vi "signalThreshold.vi"(11 "VE":dbl[](array[numeric])) -> (2 "minValue":dbl, 3 "Threshould":dbl)   [LabVIEW 2011]
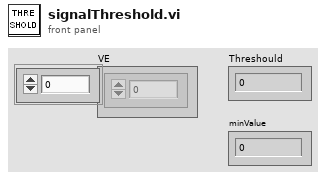
[diagram p1: front panel]
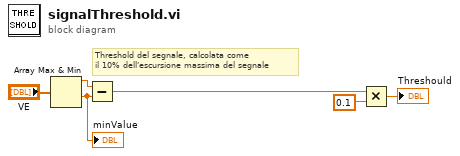
[diagram p0: block diagram]
diagram:
  # "Threshold del segnale, calcolata come\nil 10% dell'escursione massima del segnale"
  n1 = Array Max & Min(array="VE") -> (max value=w1:dbl, min value=w2:dbl)  [unwired: 2 out]
  "minValue" <- w2
  n2 = Subtract(x=w1, y=w2) -> (x-y=w3:dbl)
  n3 = Multiply(x=w3, y=0.1) -> (x*y=→"Threshould":dbl)
